vi "Fast Section Create FuncGlobal.vi"(4 "Property Values":variant[](array[variant]), 5 "Action":enum16{"Open or Add", "Close Ref"}(ring), 6 "Property names":string[](array[string]), 7 "GUID (Default Section)":string="03D3BB89-1485-13A6-56005DE6430FF8B7", 8 "error in (no error)":errorcluster, 10 "Section Name":string, 11 "Parent Ref in":T1 format="%.0x") -> (0 "error out":errorcluster, 1 "Section Ptr":T1 format="%.0x", 2 "Newly Created?":bool, 3 "Parent Ref out":T1 format="%.0x")   [LabVIEW 2011]
doc: "Creates an NI VeriStand Section faster than the built in function does (when called in a loop). The built in function opens a reference and closes it within, causing it to be realllly slow in a loop. This functional global opens the reference on first call, but then saves it for later use.\n\nMake sure you close the refernce later."
uses:
  <vilib>/NI Veristand/Custom Device API/Custom Device Item Ref.ctl
  <vilib>/NI Veristand/Custom Device API/Custom Device API.lvlib
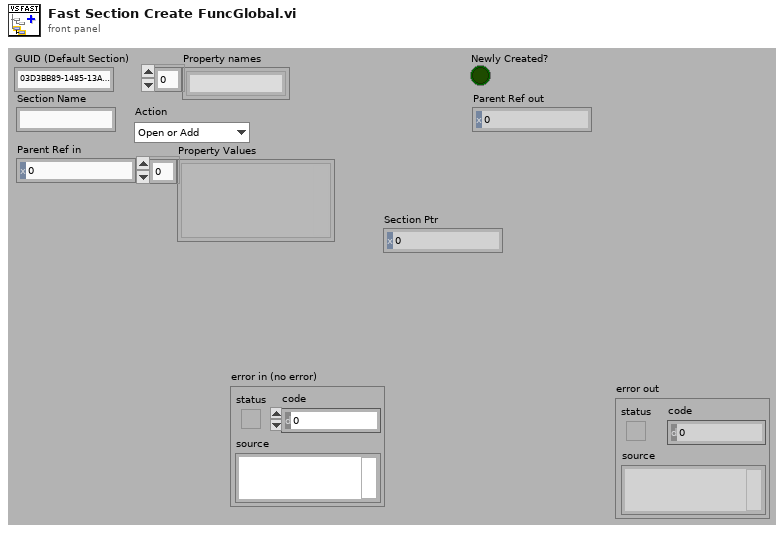
[diagram p1: front panel]
types:
  T1 = typedef "Custom Device API.lvlib/Custom Device Item Ref.ctl" = u64
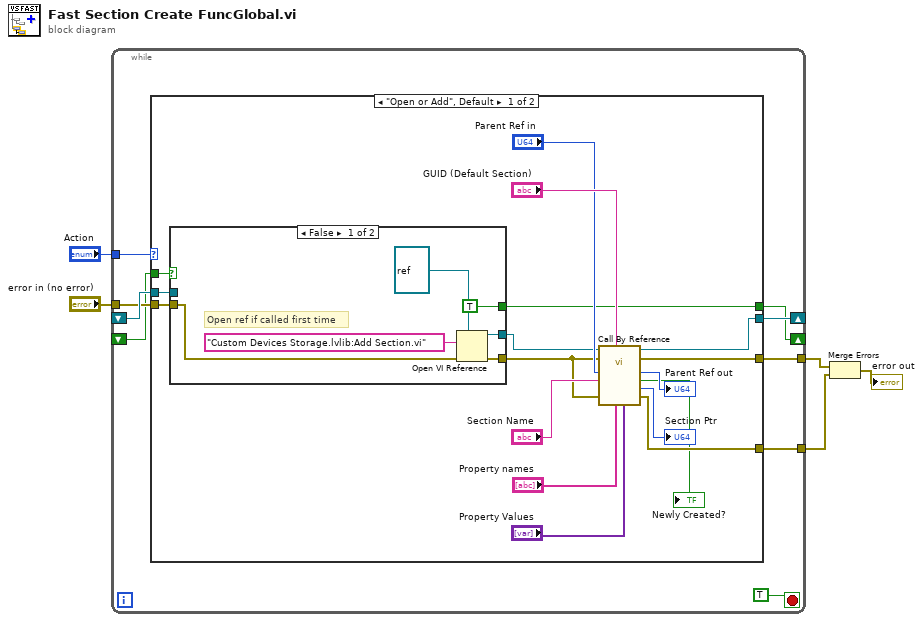
[diagram p0: block diagram]
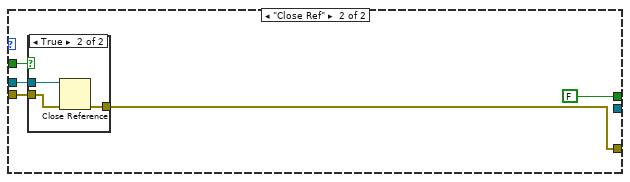
[diagram p3: hidden frame]
diagram:
  n1 = while {
    tunnel: "Action" -> [w14]
    shift-right: [w13] -> _
    shift-left: _ -> [w12]
    tunnel: "error in (no error)" -> [w11]
    tunnel: [w10] -> w2
    tunnel: [w9] -> w1
    shift-right: [w8] -> _
    shift-left: _ -> [w7]
    stop <- TRUE stop-if-true
    n2 = case shown="\"Open or Add\", Default" w14 {
      tunnel: w12 -> [w16 w45]
      tunnel: [w24 _] -> w13
      tunnel: w11 -> [w21 w44]
      tunnel: [w23 _] -> w10
      tunnel: [w22 w41] -> w9
      tunnel: [w19 FALSE] -> w8
      tunnel: w7 -> [w18 w42]
      frame "Open or Add", Default {
        n3 = case shown="False" w18 {
          selector: w18 -> [_ w38]
          tunnel: w21 -> [w36 w39]
          tunnel: [w35 w39] -> w20
          tunnel: [TRUE w38] -> w19
          tunnel: [w33 w40] -> w17
          tunnel: w16 -> [_ w40]
          frame False {
            # "Open ref if called first time"
            n4 = Open VI Reference(type specifier VI Refnum (for type only)=refnum<vi> refnum, vi path="Custom Devices Storage.lvlib:Add Section.vi", error in (no error)=w36) -> (vi reference=w33:refnum<vi>, error out=w35:errorcluster)  [unwired: 1 in, 2 out]
          }
          frame True {
            # "Don't open the ref if already open"
          }
        }
        n5 = call-by-ref "?"(reference=w17, error in=w20, "Property Values"="Property Values", "Property names"="Property names", "GUID (Default Section)"="GUID (Default Section)", 8:"error in (no error)"=w20, "Section Name"="Section Name", "Parent Ref in"="Parent Ref in") -> (reference out=w24:refnum<vi>, error out=w22:errorcluster, 0:"error out"=w23:errorcluster, "Section Ptr"=→"Section Ptr":T1, "Newly Created?"=→"Newly Created?":bool, "Parent Ref out"=→"Parent Ref out":T1)  [unwired: 2 in]
      }
      frame "Close Ref" {
        n6 = case shown="True" w42 {
          tunnel: w45 -> [_ w49]
          tunnel: w44 -> [w46 w48]
          tunnel: [w46 w47] -> w41
          frame False {
          }
          frame True {
            n7 = Close Reference(reference=w49, error in (no error)=w48) -> (error out=w47:errorcluster)
          }
        }
      }
    }
  }
  n8 = Merge Errors(w1, w2) -> (→"error out":errorcluster)
